vi "server fix fix.vi"() -> ()   [LabVIEW 2017]
uses:
  <vilib>/Analysis/Matrix/Datatypes/RealMatrix.ctl
  <vilib>/Platform/TimedLoop/XDataNode/timing_clust.ctl
  <vilib>/Platform/TimedLoop/XDataNode/nitl_modes.ctl
  <vilib>/Platform/TimedLoop/XDataNode/wakeup.ctl
  <vilib>/platform/TimedLoop/XDataNode/XDataNode.xnode
  <vilib>/Platform/TimedLoop/XDataNode/XDNodeRunTimeDep.lvlib
  <vilib>/Analysis/Matrix/NI_Matrix.lvlib
panel:
  out "appended array":T1
  in  "?":dbl[](array[numeric])
  in  "?":dbl[](array[numeric])
  in  "?":dbl[](array[numeric])
  in  "?":dbl[](array[numeric])
  in  "?":dbl[](array[numeric])
  in  "?":dbl[](array[numeric])
  in  "?":dbl[](array[numeric])
  in  "?":dbl[](array[numeric])
  out "Error":errorcluster
  out "Expected End [i-1]":i64
  out "Actual End [i-1]":i64
  out "Finished Late? [i-1]":bool
  out "Iteration Duration":i64
  out "Processor 2":i32=-2
  out "Global End Time":i64
  in  "Processor":i32=-2
  out "?":string="SERVER"
  out "BYTE WRITE FROM SERVER":i32
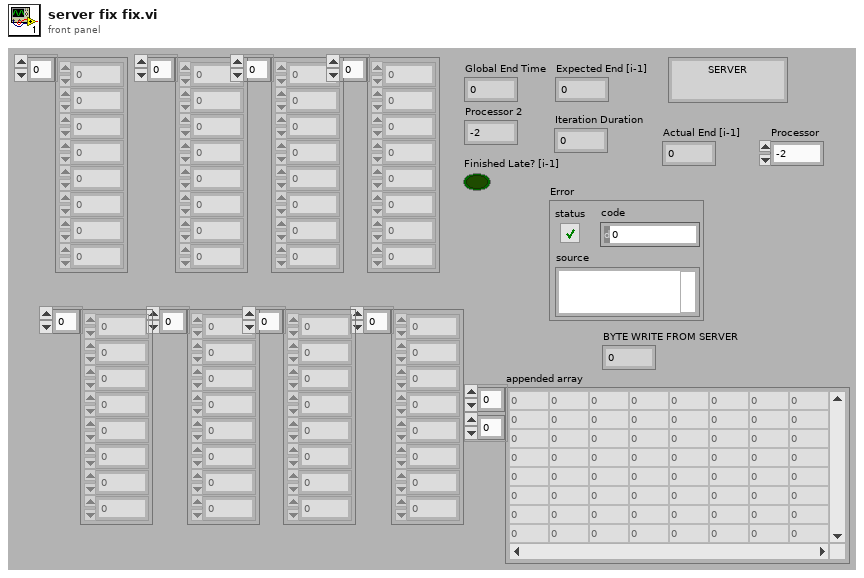
[diagram p1: front panel]
types:
  T1 = typedef "NI_Matrix.lvlib/RealMatrix.ctl" = dbl[][]
  T2 = typedef "XDNodeRunTimeDep.lvlib/timing_clust.ctl" = cluster{"Expected End [f-1]":u64, "Actual End [f-1]":u64, "Finished Late? [f-1]":bool, "Expected End [i-1]":u64, "Actual End [i-1]":u64, "Finished Late? [i-1]":bool, "Expected Start [i]":u64, "Actual Start [i]":u64, "Expected Start [f]":u64, "Actual Start [f]":u64, "Source Name":string, "Structure Name":string, "Period":i64, "Deadline":i64, "Offset":i64, "Start":i64, "Priority":i32, "Timeout":i32, "Mode":T3, "Wakeup Reason":T4, "Error":errorcluster, "Source Type":string, "Secondary Source Type":string, "Global End Time":u64, "Global Start Time":u64, "Frame Duration":u64, "Iteration Duration":u64, "Assigned CPU":i32, "I/O Scan Engine Mode":u32}
  T3 = typedef "XDNodeRunTimeDep.lvlib/nitl_modes.ctl" = enum32{"No Change", "Process missed periods, maintain original phase", "Discard missed periods, maintain original phase", "Process missed periods, ignore original phase", "Discard missed periods, ignore original phase"}
  T4 = typedef "XDNodeRunTimeDep.lvlib/wakeup.ctl" = enum32{"Normal", "Aborted", "Asynchronous wakeup", "Timing source error", "Timed loop error", "Timeout"}
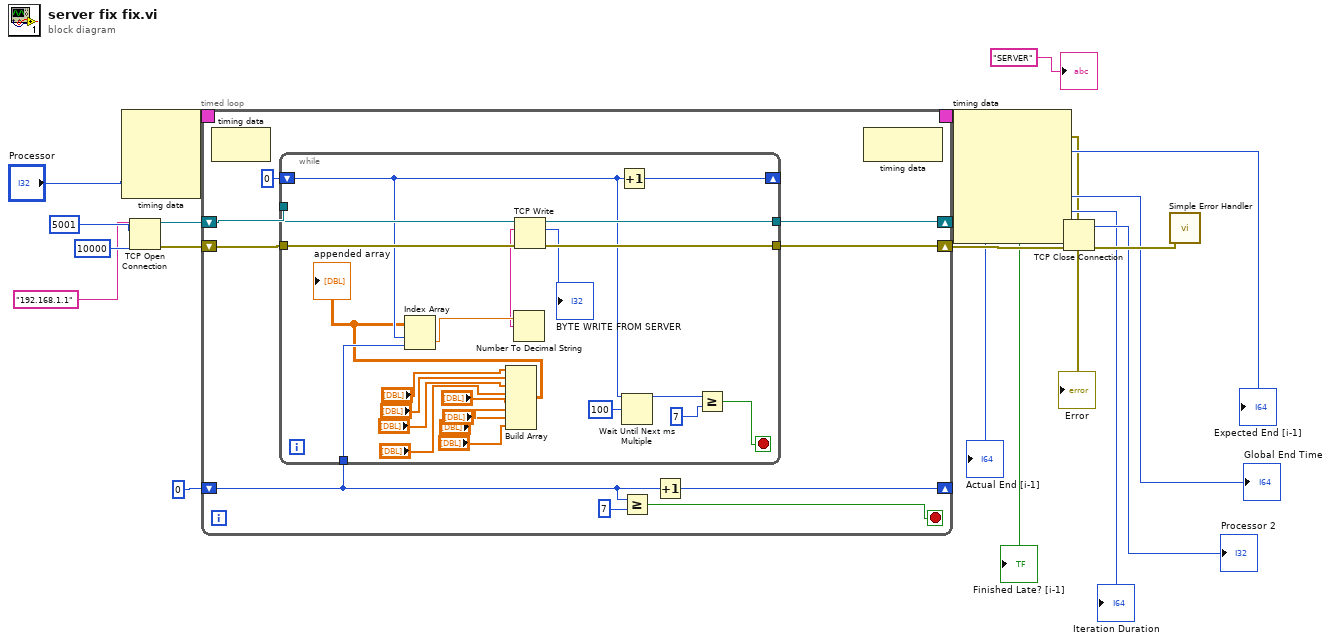
[diagram p0: block diagram]
diagram:
  n1 = node-c288("Processor") -> (w11:T2)  [unwired: 3 in]
  n2 = TCP Open Connection(address="192.168.1.1", remote port or service name=u16 5001, timeout ms (60000)=10000) -> (connection ID=w18:refnum<k5>, error out=w17:errorcluster)  [unwired: 2 in]
  n3 = timed-loop {
    shift-right: [w27] -> w15
    shift-left: w18 -> [w29]
    shift-right: [w26] -> w14
    shift-left: w17 -> [w28]
    shift-right: [w24] -> _
    shift-left: 0 -> [w21]
    timing: w11 -> [_]
    timing-out: [_] -> w10
    stop <- w22 stop-if-true
    n4 = node-c288() -> ()  [unwired: 1 in, 1 out]
    n5 = while {
      tunnel: w29 -> [w53]
      tunnel: w28 -> [w52]
      tunnel: [w51] -> w27
      tunnel: [w50] -> w26
      shift-right: [w45] -> _
      shift-left: 0 -> [w44]
      tunnel: w21 -> [w41]
      stop <- w42 stop-if-true
      n6 = Build Array("?", "?", "?", "?", "?", "?", "?", "?") -> (w32:T1)
      "appended array" <- w32
      n7 = Index Array(array=w32, index (row)=w44, index (col)=w41) -> (element=w48:dbl)
      n8 = Number To Decimal String(number=w48) -> (decimal integer string=w47:string)  [unwired: 1 in]
      n9 = TCP Write(connection ID=w53, data in=w47, error in (no error)=w52) -> (connection ID out=w51:refnum<k5>, bytes written=→"BYTE WRITE FROM SERVER":i32, error out=w50:errorcluster)  [unwired: 1 in]
      n10 = Increment(x=w44) -> (x+1=w45:i32)
      n11 = Wait Until Next ms Multiple(millisecond multiple=u32 100) -> ()  [unwired: 1 out]
      n12 = Greater Or Equal?(x=w44, y=7) -> (x >= y?=w42:bool)
    }
    n13 = Greater Or Equal?(x=w21, y=7) -> (x >= y?=w22:bool)
    n14 = Increment(x=w21) -> (x+1=w24:i32)
    n15 = node-c288() -> ()  [unwired: 1 in, 1 out]
  }
  n16 = node-c288(w10) -> (→"Error":errorcluster, →"Expected End [i-1]":i64, →"Actual End [i-1]":i64, →"Finished Late? [i-1]":bool, →"Global End Time":i64, →"Iteration Duration":i64, →"Processor 2":i32)
  n17 = TCP Close Connection(connection ID=w15, error in (no error)=w14) -> (error out=w16:errorcluster)  [unwired: 1 in, 1 out]
  n18 = call <vilib>:"Simple Error Handler.vi"("error in (no error)"=w16) -> ()  [unwired: 4 in, 5 out]
  "?" <- "SERVER"
